vi "Write_Characters_To_File.vi"(0 "file path (dialog if empty)":path, 1 "advisory dialog? (display:T)":bool=TRUE, 2 "character string":string, 3 "append to file? (new file:F)":bool, 4 "Lock File":bool) -> (8 "mark after write (bytes)":i32)   [LabVIEW 2015]
doc: "Writes a character string to a new byte stream file or appends the string to an existing file. The VI opens or creates the file beforehand and closes it afterwards.\n\nfile path is the path name of the file. If file path is empty (default value) or is Not A Path, the VI displays a File dialog box from which you can select a file. Error 43 occurs if the user cancels the dialog. \n\ncharacter string is the data the VI writes to the file.\n\nappend to file? Set to TRUE if you want to append the data to a existing file; you can also set it TRUE to write to a new file. Set to FALSE (default value) if you want to write the data to a new file or to replace an existing file.\n\nnew file path is the path of the file to which the VI wrote data. You can use this output to determine the path of a file that you open using dialog. new file path returns Not A Path if the user selects Cancel from the dialog box."
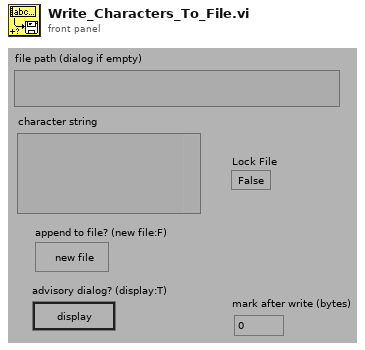
[diagram p1: front panel]
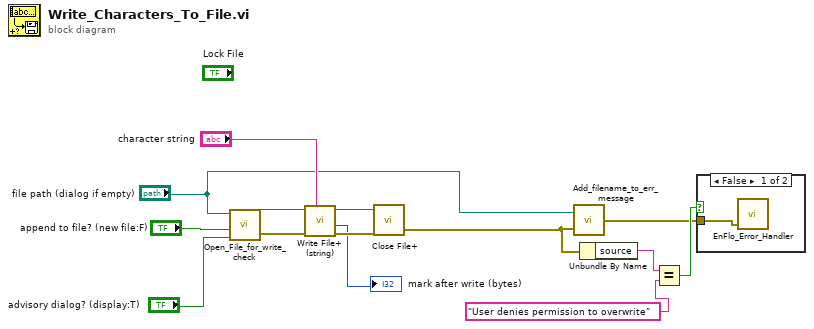
[diagram p0: block diagram]
diagram:
  n1 = call "Open_File_for_write_check.vi"("advisory dialog? (display:T)"="advisory dialog? (display:T)", "append to file? (new file:F)"="append to file? (new file:F)", "file path"="file path (dialog if empty)") -> ("error out"=w9:errorcluster, "refnum"=w10:refnum<file>)  [unwired: 7 out]
  n2 = call <vilib>:"Write File+ (string).vi"("string"="character string", "error in (no error)"=w9, "refnum"=w10) -> ("error out"=w14:errorcluster, "mark after write (bytes)"=→"mark after write (bytes)":i32, "dup refnum"=w13:refnum<file>)  [unwired: 2 in, 2 out]
  n3 = call <vilib>:"Close File+.vi"("error in (no error)"=w14, "refnum"=w13) -> ("error out"=w5:errorcluster)  [unwired: 5 out]
  n4 = call "Add_filename_to_err_message.vi"("error in (no error)"=w5, "Path"="file path (dialog if empty)") -> ("error out"=w1:errorcluster)
  n5 = Unbundle By Name(w5) -> ("source"=w3:string)
  n6 = Equal?(x=w3, y="User denies permission to overwrite") -> (x = y?=w2:bool)
  n7 = case shown="False" w2 {
    tunnel: w1 -> [w15 _]
    frame False {
      n8 = call "EnFlo_Error_Handler.vi"("error in (no error)"=w15) -> ()  [unwired: 2 in, 3 out]
    }
    frame True {
    }
  }
